vi "accum-1D-array-to-sizeN-and-pop.vi"(4 "flush":bool, 6 "Nsize":i32, 8 "new-data-in":dbl[](array[numeric]), 11 "old-data-in":dbl[](array[numeric])) -> (0 "popped-data":dbl[](array[numeric]), 1 "new-data-ready":bool, 3 "old-data-out":dbl[](array[numeric]))   [LabVIEW 2017]
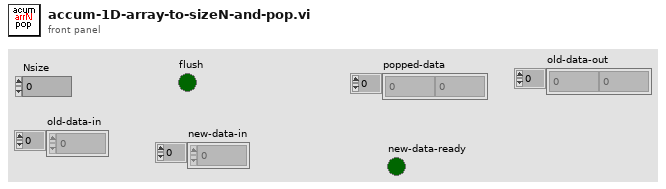
[diagram p1: front panel]
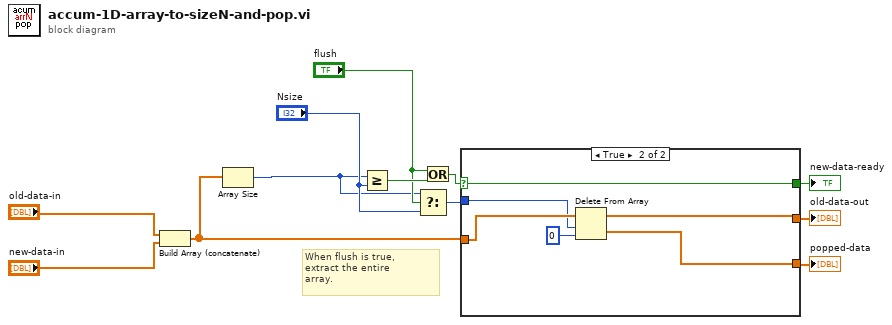
[diagram p0: block diagram]
diagram:
  # "When flush is true,\nextract the entire \narray."
  n1 = Build Array (concatenate)("old-data-in", "new-data-in") -> (w12:dbl[])
  n2 = Array Size(array=w12) -> (size(s)=w1:i32)
  n3 = Greater Or Equal?(x=w1, y="Nsize") -> (x >= y?=w4:bool)
  n4 = Select(t=w1, s="flush", f="Nsize") -> (s? t:f=w6:i32)
  n5 = Or(x="flush", y=w4) -> (x .or. y?=w3:bool)
  n6 = case shown="True" w3 {
    selector: w3 -> [w13 w20]
    tunnel: [w14 w16] -> w8
    tunnel: w12 -> [w14 w19]
    tunnel: [w13 w20] -> w10
    tunnel: w6 -> [_ w17]
    tunnel: [_ w15] -> w11
    frame False {
    }
    frame True {
      n7 = Delete From Array(array=w19, length=w17, index=0) -> (deleted portion=w15:dbl[], array with subset deleted=w16:dbl[])
    }
  }
  "popped-data" <- w11
  "new-data-ready" <- w10
  "old-data-out" <- w8
